vi "main.vi"   [LabVIEW 2017, in "NullPatternDemo.lvclass"]
uses:
  NullPatternDemo.lvclass
  CustomerFactory Class/CustomerFactory.lvclass
  ConsoleOut/Print Options.ctl
  NullCustomer Class/NullCustomer.lvclass
  C:/Users/fflores/Documents/LabVIEW-Open-Projects/LabIVEW OOP Design Patterns/Null Object Pattern/AbstractCustomer Class/AbstractCustomer.lvclass
  RealCustomer Class/RealCustomer.lvclass
  RealCustomer Class/RealCustomer.vi
  AbstractCustomer Class/AbstractCustomer.lvclass
types:
  T1 = typedef "Print Options.ctl" = enum16{"Create", "Get Reference", "Print", "Print Header", "Close"}
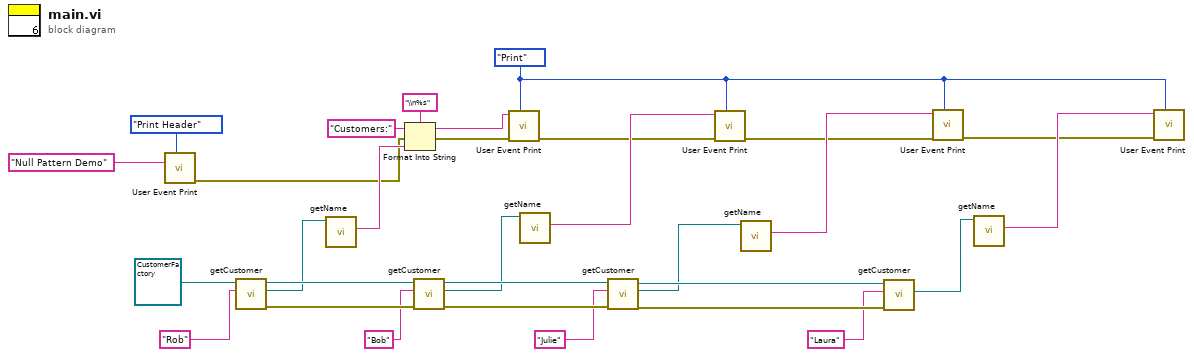
[diagram p0: block diagram]
diagram:
  w4 = Print_Options."Print" ("Options")
  n1 = call "User Event Print.vi"("Options"=Print_Options."Print Header", "String to Print"="Null Pattern Demo") -> ("error out"=w2:errorcluster)  [unwired: 8 in, 1 out]
  n2 = call "getCustomer.vi"("name"="Rob", "CustomerFactory in"=refnum<class "CustomerFactory.lvclass"> refnum ("CustomerFactory.lvclass")) -> ("error out"=w28:errorcluster, "AbstractCustomer.lvclass"=w17:refnum<class "AbstractCustomer.lvclass">, "CustomerFactory out"=w29:refnum<class "CustomerFactory.lvclass">)  [unwired: 7 in]
  n3 = call-dynamic "getName.vi"("AbstractCustomer in"=w17) -> ("name"=w18:string)  [unwired: 8 in, 2 out]
  n4 = Format Into String(format string="\\n%s", initial string="Customers:", error in=w2, w18) -> (resulting string=w7:string, error out=w9:errorcluster)
  n5 = call "getCustomer.vi"("error in (no error)"=w28, "name"="Bob", "CustomerFactory in"=w29) -> ("error out"=w26:errorcluster, "AbstractCustomer.lvclass"=w16:refnum<class "AbstractCustomer.lvclass">, "CustomerFactory out"=w27:refnum<class "CustomerFactory.lvclass">)  [unwired: 6 in]
  n6 = call "User Event Print.vi"("Options"=w4, "error in (no error)"=w9, "String to Print"=w7) -> ("error out"=w8:errorcluster)  [unwired: 7 in, 1 out]
  n7 = call-dynamic "getName.vi"("AbstractCustomer in"=w16) -> ("name"=w15:string)  [unwired: 8 in, 2 out]
  n8 = call "getCustomer.vi"("error in (no error)"=w26, "name"="Julie", "CustomerFactory in"=w27) -> ("error out"=w24:errorcluster, "AbstractCustomer.lvclass"=w14:refnum<class "AbstractCustomer.lvclass">, "CustomerFactory out"=w25:refnum<class "CustomerFactory.lvclass">)  [unwired: 6 in]
  n9 = call "User Event Print.vi"("Options"=w4, "error in (no error)"=w8, "String to Print"=w15) -> ("error out"=w6:errorcluster)  [unwired: 7 in, 1 out]
  n10 = call-dynamic "getName.vi"("AbstractCustomer in"=w14) -> ("name"=w13:string)  [unwired: 8 in, 2 out]
  n11 = call "getCustomer.vi"("error in (no error)"=w24, "name"="Laura", "CustomerFactory in"=w25) -> ("AbstractCustomer.lvclass"=w12:refnum<class "AbstractCustomer.lvclass">)  [unwired: 6 in, 2 out]
  n12 = call "User Event Print.vi"("Options"=w4, "error in (no error)"=w6, "String to Print"=w13) -> ("error out"=w5:errorcluster)  [unwired: 7 in, 1 out]
  n13 = call-dynamic "getName.vi"("AbstractCustomer in"=w12) -> ("name"=w11:string)  [unwired: 8 in, 2 out]
  n14 = call "User Event Print.vi"("Options"=w4, "error in (no error)"=w5, "String to Print"=w11) -> ()  [unwired: 7 in, 2 out]
